vi "Dialog_EditFormulas.vi"(8 "error in (no error)":errorcluster, 11 "launcher":refnum<class "launcher.lvclass">) -> (0 "error out":errorcluster)   [LabVIEW 2021, in "launcher.lvclass"]
uses:
  launcher.lvclass
  C:/Program Files (x86)/National Instruments/LabVIEW 2021/user.lib/S2 Labs/Module Framework/Modules/Base/Module.lvclass
  <userlib>/S2 Labs/Queued State Machine/TypeDefs/Queue Message.ctl
  <userlib>/S2 Labs/Queued State Machine/TypeDefs/States.ctl
  <userlib>/S2 Labs/Module Framework/Modules/Base/Module.lvclass/Module.ctl
  <userlib>/S2 Labs/Queued State Machine/QSM.lvclass/QSM.ctl
  <userlib>/S2 Labs/Queued State Machine/Callback Notifier/Callback Notifier.lvclass/Callback Notifier.ctl
  <userlib>/S2 Labs/Module Framework/Modules/Formulas/TypeDefs/Formula Config Element.ctl
  <userlib>/S2 Labs/CVT Toolkit/CVT.lvclass/CVT.ctl
  <vilib>/LAVA/muParser/mupExpr/mupExpr.lvclass
  <vilib>/LAVA/muParser/mupExpr/mupExpr.lvclass/mupExpr.ctl
  e3e9dbb3-798f-4662-8ad2-2efcafa2ef06.vi
  2f4164a3-385f-4925-8ffb-7f0685e2441d.vi
  408738d8-71eb-4504-8fdf-b52b68c66d6e.vi
  a5bd8fd8-7a3d-473a-a376-97eedd6874f0.vi
  5eef2af3-9d6d-494e-b222-9a4d6e3083c3.vi
  11bf041d-e9cc-4984-a70b-da3cb4fb70fe.vi
  <vilib>/LAVA/muParser/mupExpr/Eval_MultiVar_SglRes.vi
  e3e9dbb3-798f-4662-8ad2-2efcafa2ef06.vi/a5442550-30ab-4f7c-a4e8-4e040bcf3d57.vi
  <userlib>/S2 Labs/Module Framework/Modules/Base/Read Queue.vi
  e3e9dbb3-798f-4662-8ad2-2efcafa2ef06.vi/77abbf80-a0d7-431e-91bd-d2268efe8bf3.vi
  e3e9dbb3-798f-4662-8ad2-2efcafa2ef06.vi/7a27d807-84e4-485a-8ba6-289735576614.vi
  <userlib>/S2 Labs/Queued State Machine/Callback Notifier/Read Callback Notifier Ref.vi
  a5bd8fd8-7a3d-473a-a376-97eedd6874f0.vi/a5442550-30ab-4f7c-a4e8-4e040bcf3d57.vi
  a5bd8fd8-7a3d-473a-a376-97eedd6874f0.vi/77abbf80-a0d7-431e-91bd-d2268efe8bf3.vi
  a5bd8fd8-7a3d-473a-a376-97eedd6874f0.vi/7a27d807-84e4-485a-8ba6-289735576614.vi
  5eef2af3-9d6d-494e-b222-9a4d6e3083c3.vi/1553f4ce-967c-4f57-a913-5f155bf4374d.vi
  11bf041d-e9cc-4984-a70b-da3cb4fb70fe.vi/1553f4ce-967c-4f57-a913-5f155bf4374d.vi
  <vilib>/LAVA/muParser/mupExpr/SetVarVal.vi
  <vilib>/LAVA/muParser/mupLib/mupEval.vi
  <userlib>/S2 Labs/Queued State Machine/Enqueue Element.vi
  <userlib>/S2 Labs/CVT Toolkit/Read CVT DVR.vi
  <vilib>/LAVA/muParser/mupLib/mupSetVarValue.vi
  <vilib>/LAVA/muParser/mupLib/mupCheckError.vi
  <userlib>/S2 Labs/Module Framework/Modules/Base/Get Module Queues Map.vi
  <userlib>/S2 Labs/Queued State Machine/Callback Notifier/Obtain Callback Notifier.vi
  <userlib>/S2 Labs/Queued State Machine/Callback Notifier/Release Reply Notifier.vi
  <vilib>/JDP Science/JSONtext/Variant to JSON Text.vi
  <userlib>/S2 Labs/Alarms and Events Toolkit/Alarms/Set User Event.vi
  <userlib>/S2 Labs/Module Framework/Modules/Base/Get Module CVT Ref.vi
  <vilib>/Utility/error.llb/Error Cluster From Error Code.vi
  <userlib>/S2 Labs/Queued State Machine/QSM.lvclass
  <userlib>/S2 Labs/Queued State Machine/Callback Notifier/Callback Notifier.lvclass
  <vilib>/JDP Science/JSONtext/LVClass Serializer/JSONtext LVClass Serializer.lvclass
  <userlib>/S2 Labs/Module Framework/Modules/Formulas/Formulas Base.lvclass
panel:
  out "Double-clicked Row":i32
  in  "OK":bool
  in  "Cancel":bool
  in  "Tab":enum32{"Formulas List", "Edit"}(tab)
  in  "Edit":bool
  in  "Delete":bool
  in  "Add":bool
  in  "Alarms List":i32(listbox)
  in  "Insert Ch":bool
  in  "Channels":i32(listbox)
  in  "Module":string(combo)="A1 Battery Pack 1"
  out "Variables":i32(listbox)
  out "Result":dbl
  in  "TestAlarm":bool
  in  "Unit":string
  in  "Formula":string
  in  "Name":string
  out "error":errorcluster
  out "Debug Message":string
  # "Or Double-Click Item to Edit..."
  # "Edit Formula"
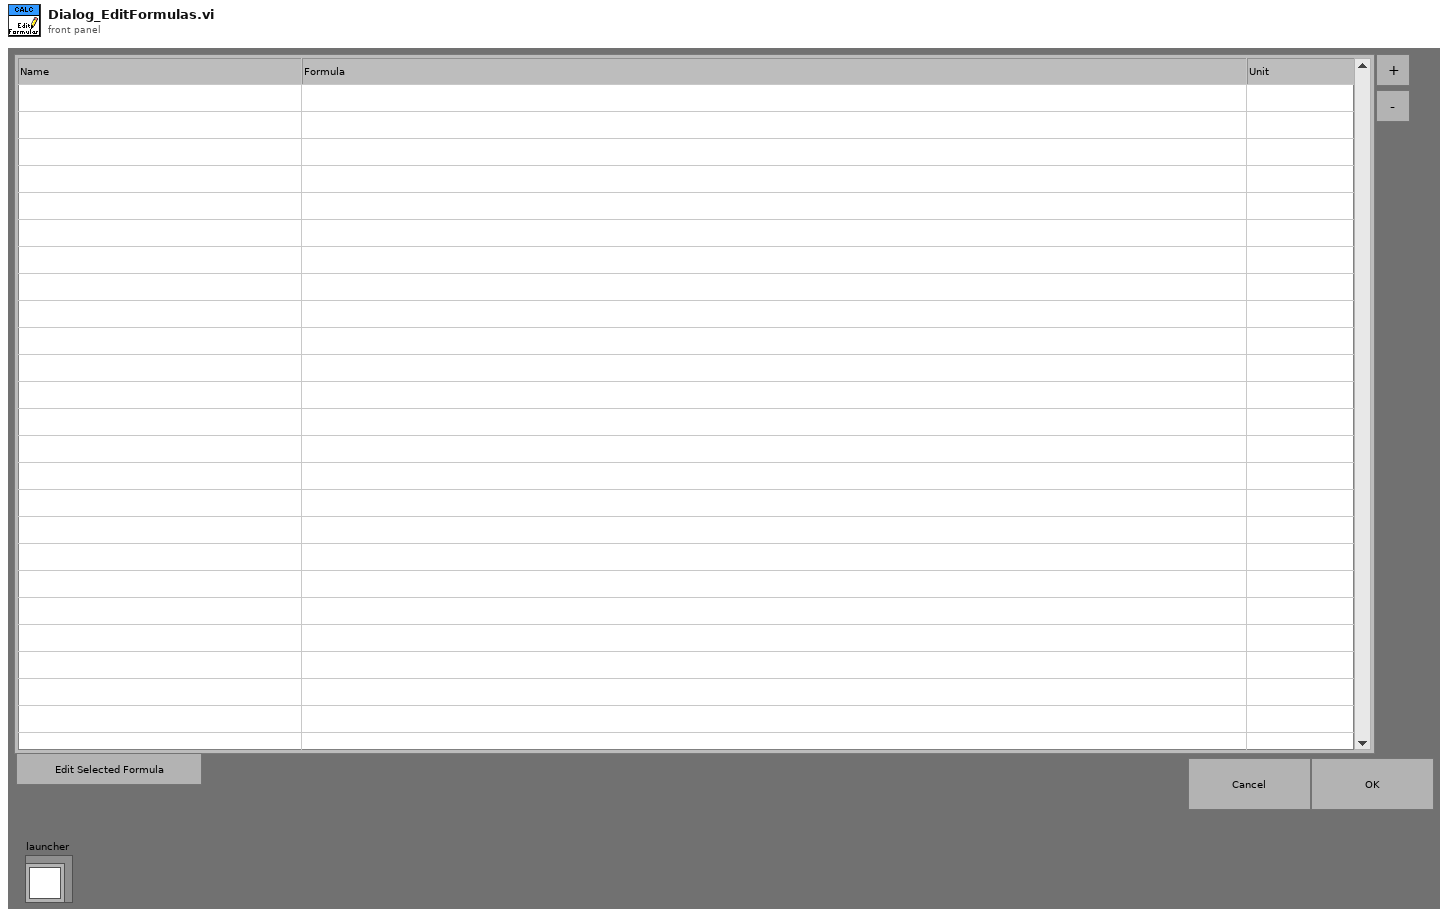
[diagram p1: front panel]
types:
  T1 = cluster{"Name":string, "Formula":string, "Unit":string}[]
  T2 = typedef "QSM.lvclass/Queue Message.ctl" = cluster{"State":T3, "Command":string, "Parameter":variant}
  T3 = typedef "QSM.lvclass/States.ctl" = enum16{"Waiting", "Init", "ExecCMD", "Read Config", "Write Config", "Launch", "Connect", "Recovery", "Clean Up", "Exit"}
  T4 = typedef "Formulas Base.lvclass/Formula Config Element.ctl" = cluster{"Name":string, "Formula":string, "Unit":string}
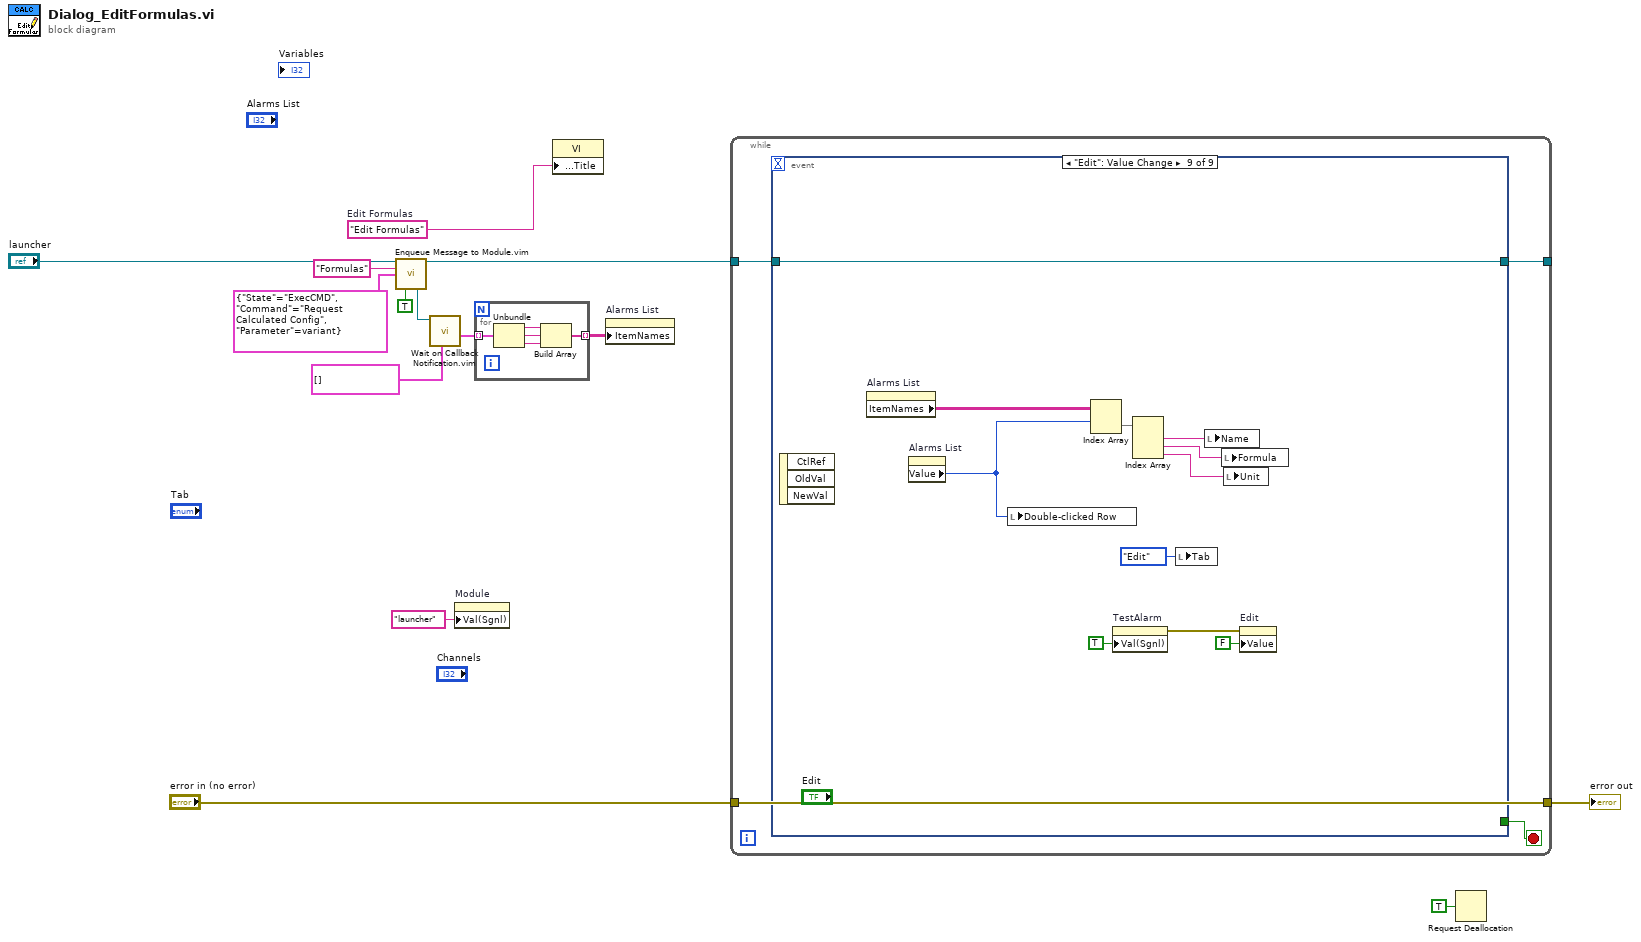
[diagram p0: block diagram]
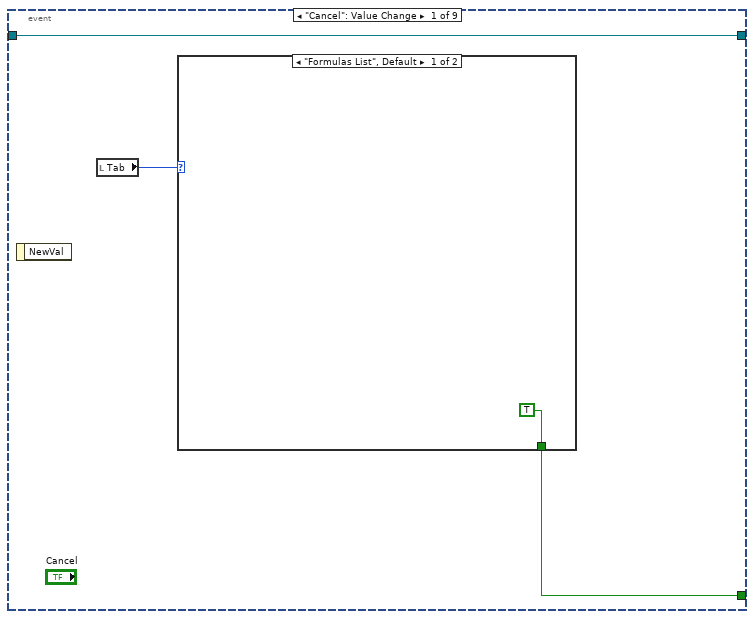
[diagram p2: hidden frame]
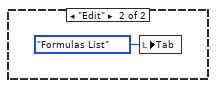
[diagram p3: hidden frame]
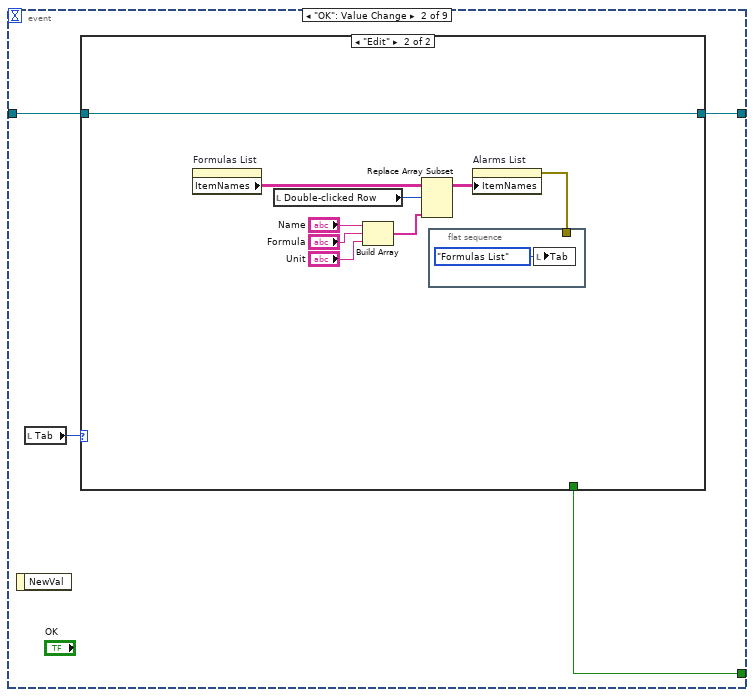
[diagram p4: hidden frame]
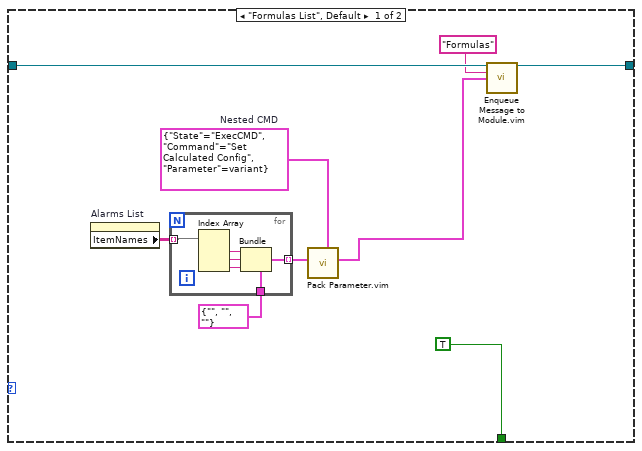
[diagram p5: hidden frame]
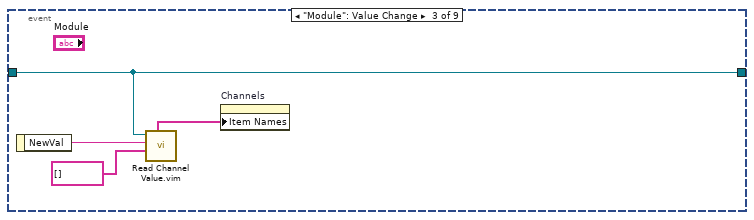
[diagram p6: hidden frame]
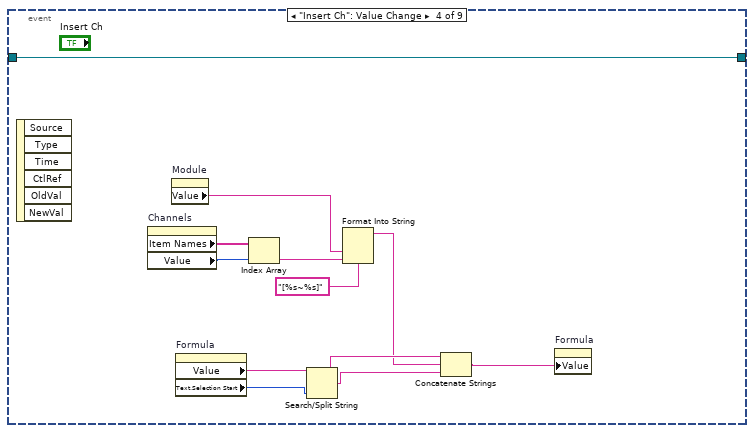
[diagram p7: hidden frame]
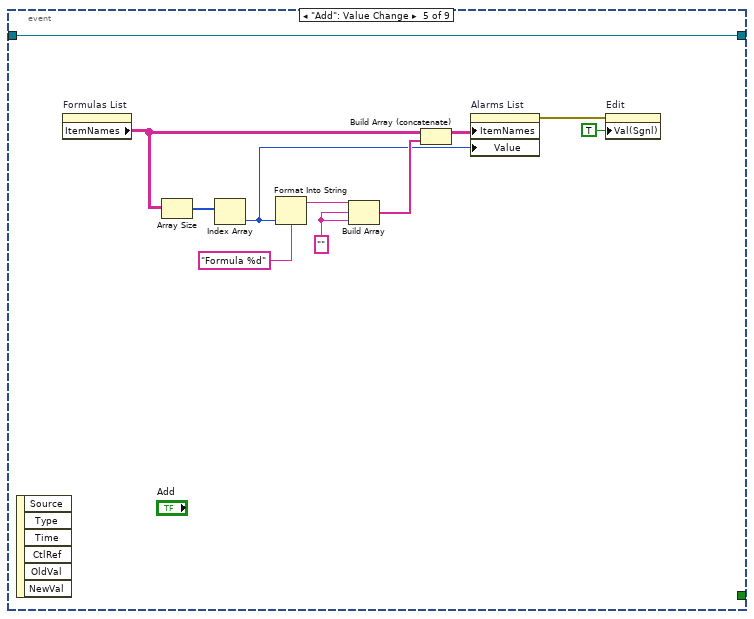
[diagram p8: hidden frame]
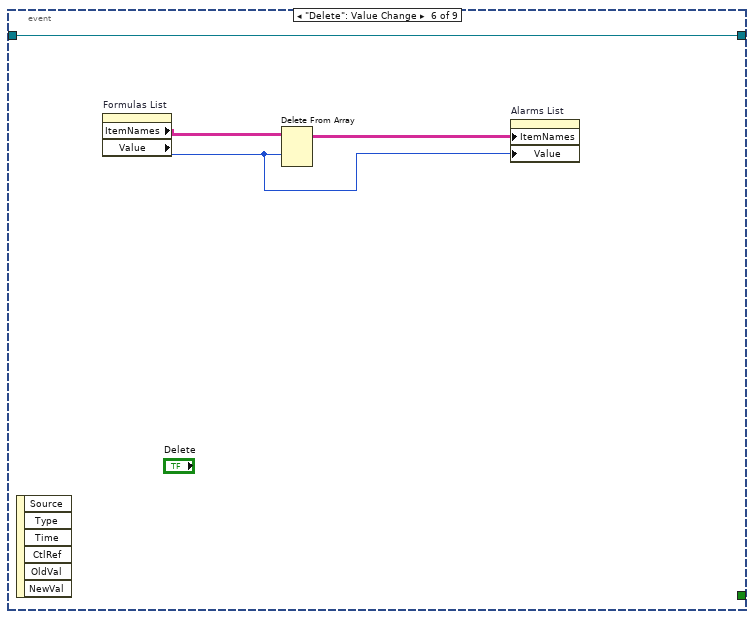
[diagram p9: hidden frame]
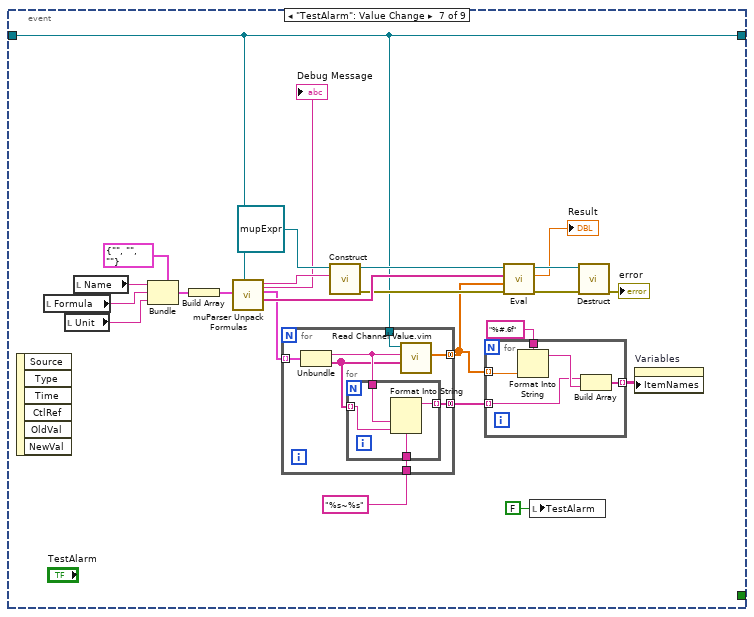
[diagram p10: hidden frame]
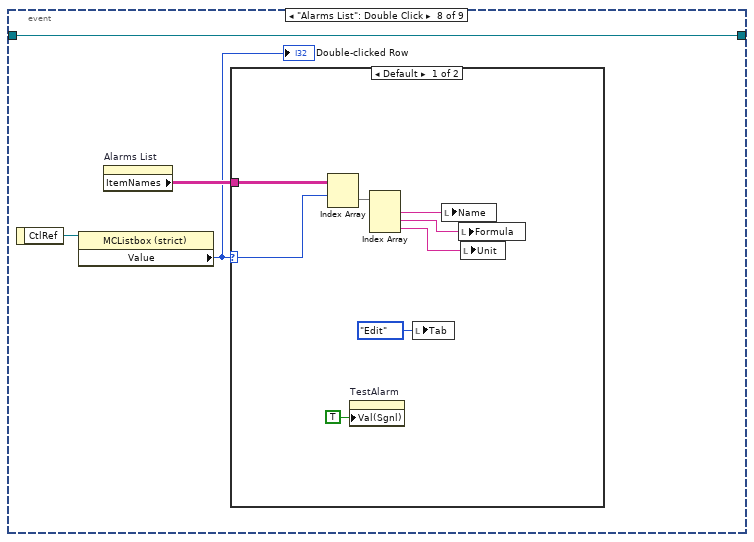
[diagram p11: hidden frame]
diagram:
  w9 = "Edit Formulas"  # Edit Formulas
  n1 = call "Enqueue Message to Module.vim"("Module in"="launcher", "Module Name (self)"="Formulas", "Message"=T2 {"State"=enum."ExecCMD", "Command"="Request Calculated Config", "Parameter"=variant}, "Request Callback Notification? (F)"=TRUE) -> ("Module out"=w10:refnum<class "launcher.lvclass">, "Callback Notifier"=w5:refnum<class "Callback Notifier.lvclass">)  [unwired: 6 in, 4 out]
  n2 = call "Wait on Callback Notification.vim"("type (string)"=T1 [] ("Cluster"), "Callback Notifier in"=w5) -> ("notification"=w2:T1)  [unwired: 6 in, 3 out]
  n3 = property on="Module" class="CmbBox"("Val(Sgnl)"="launcher" ("Value (Signaling)")) -> ()  [unwired: 2 in, 2 out]
  n4 = for {
    tunnel: w2 -> [w19] mode=indexing
    tunnel: [w15] -> w3 mode=indexing
    n5 = Unbundle(w19) -> ("Name"=w18:string, "Formula"=w17:string, "Unit"=w16:string)
    n6 = Build Array(w18, w17, w16) -> (w15:string[])
  }
  n7 = property class="VI"("Front Panel.Title"=w9) -> ()  [unwired: 2 in, 2 out]
  n8 = property on="Alarms List" class="MCListbox (strict)"("ItemNames"=w3) -> ()  [unwired: 2 in, 2 out]
  n9 = while {
    tunnel: w10 -> [w21]
    tunnel: [w22] -> _
    tunnel: [w23] -> w14
    tunnel: "error in (no error)" -> [w23]
    stop <- w20 stop-if-true
    n10 = event shown="[8] \"Edit\": Value Change" {
      selector: _ -> [_ _ _ _ _ _ _ _ _]
      dyn-events: _ -> [_ _ _ _ _ _ _ _ _]
      timeout: _ -> [_ _ _ _ _ _ _ _ _]
      tunnel: [w26 w31 w60 w73 w74 w85 w96 w131 w151] -> w22
      tunnel: w21 -> [w26 w32 w60 w73 w74 w85 w96 w131 w151]
      tunnel: [w24 w30 _ _ _ _ _ _ _] -> w20
      event "Cancel": Value Change {
        n11 = event-data() -> ()  [unwired: 1 in, 1 out]
        n12 = local read "Tab"() -> (w25:enum32{"Formulas List", "Edit"})
        n13 = case shown="\"Formulas List\", Default" w25 {
          tunnel: [TRUE _] -> w24
          frame "Formulas List", Default {
          }
          frame "Edit" {
            n14 = local write "Tab"(enum32{"Formulas List", "Edit"}."Formulas List" ("Tab")) -> ()
          }
        }
      }
      event "OK": Value Change {
        n15 = event-data() -> ()  [unwired: 1 in, 1 out]
        n16 = local read "Tab"() -> (w29:enum32{"Formulas List", "Edit"})
        n17 = case shown="\"Edit\"" w29 {
          tunnel: w32 -> [w36 w56]
          tunnel: [w35 w56] -> w31
          tunnel: [TRUE _] -> w30
          frame "Formulas List", Default {
            w37 = T2 {"State"=enum."ExecCMD", "Command"="Set Calculated Config", "Parameter"=variant}  # Nested CMD
            n18 = property on="Alarms List" class="MCListbox (strict)"() -> ("ItemNames"=w41:string[][])  [unwired: 2 in, 2 out]
            n19 = for {
              tunnel: w41 -> [w47] mode=indexing
              tunnel: T4 {"Name"="", "Formula"="", "Unit"=""} ("Cluster") -> [w43]
              tunnel: [w42] -> w38 mode=indexing
              n20 = Index Array(array=w47) -> (element #1=w46:string, element #2=w45:string, element #3=w44:string)  [unwired: 3 in]
              n21 = Bundle(cluster=w43, "Name"=w46, "Formula"=w45, "Unit"=w44) -> (w42:T4)
            }
            n22 = call "Pack Parameter.vim"("Message Cluster In"=w37, "Parameter (string)"=w38) -> ("Message Cluster Out"=w34:T2)  [unwired: 9 in]
            n23 = call "Enqueue Message to Module.vim"("Module in"=w36, "Module Name (self)"="Formulas", "Message"=w34) -> ("Module out"=w35:refnum<class "launcher.lvclass">)  [unwired: 7 in, 5 out]
          }
          frame "Edit" {
            n24 = property on="Formulas List" class="MCListbox (strict)"() -> ("ItemNames"=w52:string[][])  [unwired: 2 in, 2 out]
            n25 = local read "Double-clicked Row"() -> (w50:i32)
            n26 = Build Array("Name", "Formula", "Unit") -> (w49:string[])
            n27 = Replace Array Subset(array=w52, new element=w49, index (row)=w50) -> (w51:string[][])  [unwired: 1 in]
            n28 = flat-sequence {
              tunnel: w48 -> [_]
              frame #0 {
                n29 = local write "Tab"(enum32{"Formulas List", "Edit"}."Formulas List" ("Tab")) -> ()
              }
            }
            n30 = property on="Alarms List" class="MCListbox (strict)"("ItemNames"=w51) -> (error out=w48:errorcluster)  [unwired: 2 in, 1 out]
          }
        }
      }
      event "Module": Value Change {
        n31 = event-data() -> ("NewVal"=w59:string)  [unwired: 1 in]
        n32 = call "Read Channel Value.vim"("Channel Label(s)"=string[] [], "Module"=w59, "Module in"=w60) -> ("Channel Labels*"=w58:string[])  [unwired: 2 in, 6 out]
        n33 = property on="Channels" class="LstBox (strict)"("Item Names"=w58) -> ()  [unwired: 2 in, 2 out]
      }
      event "Insert Ch": Value Change {
        n34 = event-data() -> ()  [unwired: 1 in, 6 out]
        n35 = property on="Channels" class="LstBox (strict)"() -> ("Item Names"=w72:string[], "Value"=w71:i32)  [unwired: 2 in, 2 out]
        n36 = property on="Module" class="CmbBox"() -> ("Value"=w68:string)  [unwired: 2 in, 2 out]
        n37 = property on="Formula" class="Str"() -> ("Value"=w67:string, "Text.Selection Start"=w66:u32)  [unwired: 2 in, 2 out]
        n38 = Index Array(array=w72, index=w71) -> (element=w69:string)
        n39 = Search/Split String(string=w67, offset (0)=w66) -> (substring before match=w65:string, match + rest of string=w64:string)  [unwired: 1 in, 1 out]
        n40 = Format Into String(format string="[%s~%s]", w68, w69) -> (resulting string=w63:string)  [unwired: 2 in, 1 out]
        n41 = Concatenate Strings(w65, w63, w64) -> (w62:string)
        n42 = property on="Formula" class="Str"("Value"=w62) -> ()  [unwired: 2 in, 2 out]
      }
      event "Add": Value Change {
        w81 = ""
        n43 = event-data() -> ()  [unwired: 1 in, 6 out]
        n44 = property on="Formulas List" class="MCListbox (strict)"() -> ("ItemNames"=w80:string[][])  [unwired: 2 in, 2 out]
        n45 = Array Size(array=w80) -> (size(s)=w84:i32[])
        n46 = Index Array(array=w84) -> (element=w77:i32)  [unwired: 1 in]
        n47 = Format Into String(format string="Formula %d", w77) -> (resulting string=w82:string)  [unwired: 2 in, 1 out]
        n48 = Build Array(w82, w81, w81) -> (w78:string[])
        n49 = Build Array (concatenate)(w80, w78) -> (w79:string[][])
        n50 = property on="Alarms List" class="MCListbox (strict)"("ItemNames"=w79, "Value"=w77) -> (error out=w76:errorcluster)  [unwired: 2 in, 1 out]
        n51 = property on="Edit" class="Bool (strict)"(error in=w76, "Val(Sgnl)"=TRUE ("Value (Signaling)")) -> ()  [unwired: 1 in, 2 out]
      }
      event "Delete": Value Change {
        n52 = event-data() -> ()  [unwired: 1 in, 6 out]
        n53 = property on="Formulas List" class="MCListbox (strict)"() -> ("ItemNames"=w88:string[][], "Value"=w86:i32)  [unwired: 2 in, 2 out]
        n54 = Delete From Array(array=w88, index (row)=w86) -> (array with subset deleted=w87:string[][])  [unwired: 2 in, 1 out]
        n55 = property on="Alarms List" class="MCListbox (strict)"("ItemNames"=w87, "Value"=w86) -> ()  [unwired: 2 in, 2 out]
      }
      event "TestAlarm": Value Change {
        n56 = event-data() -> ()  [unwired: 1 in, 6 out]
        n57 = local read "Formula"() -> (w108:string)
        n58 = local read "Unit"() -> (w107:string)
        n59 = local read "Name"() -> (w109:string)
        n60 = Bundle(cluster=T4 {"Name"="", "Formula"="", "Unit"=""} ("Cluster"), "Name"=w109, "Formula"=w108, "Unit"=w107) -> (w106:T4)
        n61 = Build Array(w106) -> (w105:T4[])
        n62 = call <userlib>:"muParser Unpack Formulas.vi"("Module in"=w96, "Formulas Config"=w105) -> ("var names"=w104:string[], "CVT Requests"=w103:cluster{"module":string, "channels":string[]}[], "Formula Expressions"=w112:string, "Debug Message"=→"Debug Message":string)  [unwired: 4 in, 2 out]
        n63 = for {
          tunnel: w96 -> [w124]
          tunnel: w103 -> [w122] mode=indexing
          tunnel: [w123] -> w92 mode=concatenating
          tunnel: "%s~%s" ("format string") -> [w119]
          tunnel: [w118] -> w91 mode=concatenating
          n64 = Unbundle(w122) -> ("module"=w121:string, "channels"=w120:string[])
          n65 = for {
            tunnel: w121 -> [w127]
            tunnel: w120 -> [w126] mode=indexing
            tunnel: w119 -> [w128]
            tunnel: [w125] -> w118 mode=indexing
            n66 = Format Into String(format string=w128, w127, w126) -> (resulting string=w125:string)  [unwired: 2 in, 1 out]
          }
          n67 = call "Read Channel Value.vim"("Channel Label(s)"=w120, "Module"=w121, "Module in"=w124) -> ("value"=w123:dbl[])  [unwired: 2 in, 6 out]
        }
        n68 = call-dynamic "Construct.vi"("Expression"=w112, "muExpr in"=refnum<class "mupExpr.lvclass"> refnum) -> ("error out"=w99:errorcluster, "mupExpr out"=w102:refnum<class "mupExpr.lvclass">)  [unwired: 6 in, 2 out]
        n69 = for {
          tunnel: w92 -> [w116] mode=indexing
          tunnel: w91 -> [w114] mode=indexing
          tunnel: "%#.6f" -> [w117]
          tunnel: [w113] -> w89 mode=indexing
          n70 = Format Into String(format string=w117, w116) -> (resulting string=w115:string)  [unwired: 2 in, 1 out]
          n71 = Build Array(w114, w115) -> (w113:string[])
        }
        n72 = call-poly <vilib>:"Eval.vi"("error in (no error)"=w99, "varValues"=w92, "varNames"=w104, "muExpr in"=w102) -> ("error out"=w100:errorcluster, "Result"=→"Result":dbl, "muExpr out"=w101:refnum<class "mupExpr.lvclass">)  [unwired: 5 in]
        n73 = local write "TestAlarm"(FALSE ("TestAlarm")) -> ()
        n74 = call-dynamic "Destruct.vi"("error in (no error)"=w100, "muExpr in"=w101) -> ("error out"=→"error":errorcluster)  [unwired: 9 in]
        n75 = property on="Variables" class="MCListbox (strict)"("ItemNames"=w89) -> ()  [unwired: 2 in, 2 out]
      }
      event "Alarms List": Double Click {
        n76 = event-data() -> ("CtlRef"=w132:refnum<vi>)  [unwired: 1 in]
        n77 = property class="MCListbox (strict)"(reference=w132) -> ("Value"=w129:i32)  [unwired: 1 in, 2 out]
        "Double-clicked Row" <- w129
        n78 = property on="Alarms List" class="MCListbox (strict)"() -> ("ItemNames"=w130:string[][])  [unwired: 2 in, 2 out]
        n79 = case shown="Default" w129 {
          selector: w129 -> [w134 _]
          tunnel: w130 -> [w140 _]
          frame Default {
            n80 = Index Array(array=w140, index (row)=w134) -> (element=w139:string[])  [unwired: 1 in]
            n81 = property on="TestAlarm" class="Bool (strict)"("Val(Sgnl)"=TRUE ("Value (Signaling)")) -> ()  [unwired: 2 in, 2 out]
            n82 = Index Array(array=w139) -> (element #1=w138:string, element #2=w137:string, element #3=w136:string)  [unwired: 3 in]
            n83 = local write "Tab"(enum32{"Formulas List", "Edit"}."Edit" ("Tab")) -> ()
            n84 = local write "Name"(w138) -> ()
            n85 = local write "Formula"(w137) -> ()
            n86 = local write "Unit"(w136) -> ()
          }
          frame ..-1 {
          }
        }
      }
      event "Edit": Value Change {
        n87 = event-data() -> ()  [unwired: 1 in, 3 out]
        n88 = property on="Alarms List" class="MCListbox (strict)"() -> ("ItemNames"=w150:string[][])  [unwired: 2 in, 2 out]
        n89 = property on="Alarms List" class="MCListbox (strict)"() -> ("Value"=w143:i32)  [unwired: 2 in, 2 out]
        n90 = local write "Double-clicked Row"(w143) -> ()
        n91 = Index Array(array=w150, index (row)=w143) -> (element=w149:string[])  [unwired: 1 in]
        n92 = property on="TestAlarm" class="Bool (strict)"("Val(Sgnl)"=TRUE ("Value (Signaling)")) -> (error out=w142:errorcluster)  [unwired: 2 in, 1 out]
        n93 = Index Array(array=w149) -> (element #1=w148:string, element #2=w147:string, element #3=w146:string)  [unwired: 3 in]
        n94 = local write "Tab"(enum32{"Formulas List", "Edit"}."Edit" ("Tab")) -> ()
        n95 = local write "Name"(w148) -> ()
        n96 = local write "Formula"(w147) -> ()
        n97 = local write "Unit"(w146) -> ()
        n98 = property on="Edit" class="Bool (strict)"(error in=w142, "Value"=FALSE ("Edit")) -> ()  [unwired: 1 in, 2 out]
      }
    }
  }
  "error out" <- w14
  n99 = Request Deallocation(TRUE ("flag")) -> ()
